vi "U32toU8array.vi"(1 "x":u32=47735 format="%x") -> (0 "ArrayU8":u8[](array[numeric])=[119, 186, 0, 0] format="%x")   [LabVIEW 2015, in "VIPM2.lvlib"]
uses:
  VIPM2.lvlib
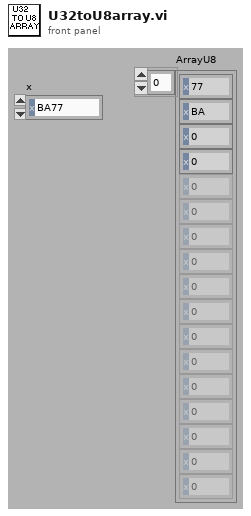
[diagram p1: front panel]
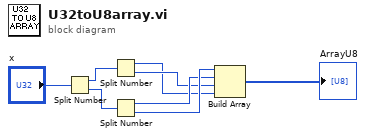
[diagram p0: block diagram]
diagram:
  n1 = Split Number(x="x") -> (hi(x)=w8:u16, lo(x)=w7:u16)
  n2 = Split Number(x=w8) -> (hi(x)=w3:u8, lo(x)=w4:u8)
  n3 = Split Number(x=w7) -> (hi(x)=w5:u8, lo(x)=w6:u8)
  n4 = Build Array "Build Array"(w6, w5, w4, w3) -> (→"ArrayU8":u8[])
